vi "midiInTranslateEvent.vi"(11 "status":i32 format="%.0x") -> (2 "Channel":i32, 3 "Message Type":T1)   [LabVIEW 2020, in "midi.lvclass"]
uses:
  midi.lvclass
  midi.lvclass/midi.ctl
  shared/midi message type.ctl
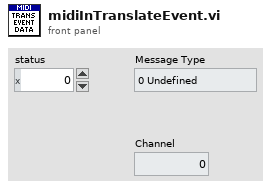
[diagram p1: front panel]
types:
  T1 = typedef "midi message type.ctl" = enum8{"0 Undefined", "1 Undefined", "2 Undefined", "3 Undefined", "4 Undefined", "5 Undefined", "6 Undefined", "7 Undefined", "Note Off", "Note On", "Polyphonic Key Pressure", "Control Change", "Program Change", "Channel Pressure", "Pitch Bend", "System Message"}
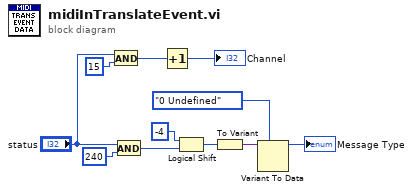
[diagram p0: block diagram]
diagram:
  n1 = And(x="status", y=15) -> (x .and. y?=w6:i32)
  n2 = And(x="status", y=240) -> (x .and. y?=w10:i32)
  n3 = Increment(x=w6) -> (x+1=→"Channel":i32)
  n4 = Logical Shift(y=i16 -4, x=w10) -> (x << y=w2:i32)
  n5 = To Variant(anything=w2) -> (Variant=w4:variant)
  n6 = Variant To Data(type=midi_message_type."0 Undefined" ("Message Type"), Variant=w4) -> (data=→"Message Type":T1)  [unwired: 1 in, 1 out]
